vi "Select Players Dialog-old.vi"(8 "error in (no error)":errorcluster, 11 "Reversi in":refnum<class "Reversi.lvclass">) -> (0 "error out":errorcluster, 3 "Reversi out":refnum<class "Reversi.lvclass">)   [LabVIEW 2021, in "Reversi.lvlib" / "Reversi.lvclass"]
uses:
  Reversi.lvclass
  Reversi.lvclass/Reversi.ctl
  aa9f3d6a-4b9f-455d-bcc5-b1d428e522bf.vi
  edd00b8c-893c-4bab-b4e2-fb96aafeb1a1.vi
  <vilib>/Comparison/Equal/Equal Functor/Equal Functor.lvclass
panel:
  in  "White":string(combo)
  in  "Black":string(combo)
  in  "Start":bool
  # "Choose Players"
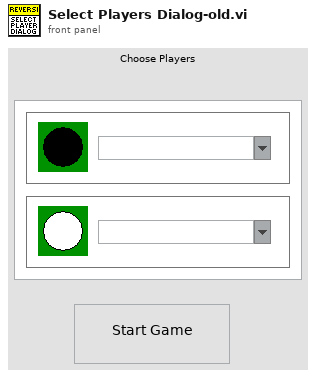
[diagram p1: front panel]
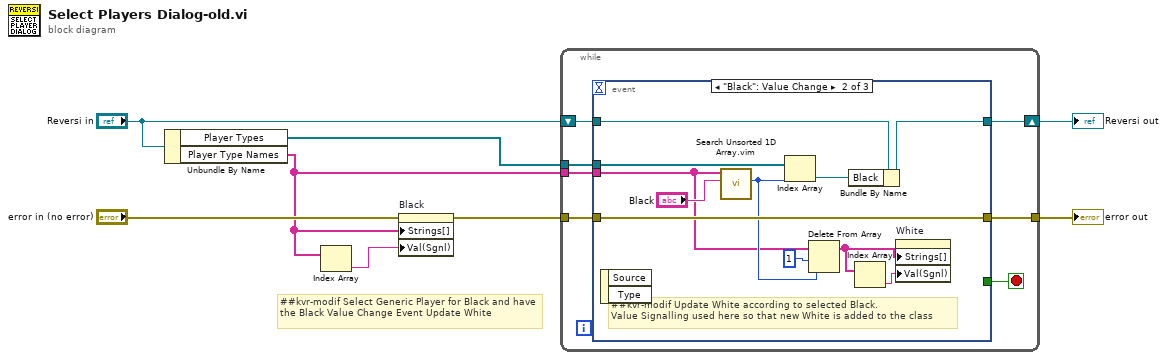
[diagram p0: block diagram]
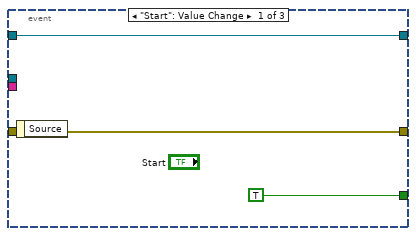
[diagram p2: hidden frame]
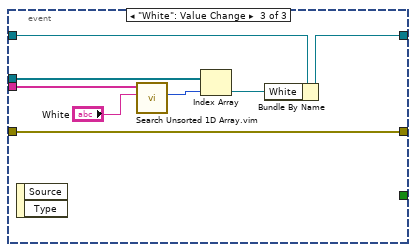
[diagram p3: hidden frame]
diagram:
  # "##kvr-modif Select Generic Player for Black and have the Black Value Change Event Update White"
  n1 = Unbundle By Name("Reversi in") -> ("Player Types"=w4:refnum<class "Player.lvclass">[], "Player Type Names"=w2:string[])
  n2 = Index Array(array=w2) -> (element=w1:string)  [unwired: 1 in]
  n3 = property on="Black" class="CmbBox"(error in="error in (no error)", "Strings[]"=w2, "Val(Sgnl)"=w1) -> (error out=w7:errorcluster)  [unwired: 1 in, 1 out]
  n4 = while {
    shift-right: [w13] -> w8
    shift-left: "Reversi in" -> [w15]
    tunnel: w4 -> [w11]
    tunnel: w2 -> [w12]
    tunnel: w7 -> [w10]
    tunnel: [w9] -> w5
    stop <- w14 stop-if-true
    n5 = event shown="[1] \"Black\": Value Change" {
      selector: _ -> [_ _ _]
      dyn-events: _ -> [_ _ _]
      timeout: _ -> [_ _ _]
      tunnel: w15 -> [w18 w26 w33]
      tunnel: [TRUE _ _] -> w14
      tunnel: [w18 w27 w34] -> w13
      tunnel: w12 -> [_ w19 w37]
      tunnel: w11 -> [_ w28 w36]
      tunnel: w10 -> [w16 w24 w30]
      tunnel: [w16 w24 w30] -> w9
      event "Start": Value Change {
        n6 = event-data() -> ()  [unwired: 1 in, 1 out]
      }
      event "Black": Value Change {
        # "##kvr-modif Update White according to selected Black.\nValue Signalling used here so that new White is added to the class"
        n7 = event-data() -> ()  [unwired: 1 in, 2 out]
        n8 = call "Search Unsorted 1D Array.vim"("element"="Black", "unsorted 1D array"=w19) -> ("index of element"=w20:i32)  [unwired: 9 in]
        n9 = Index Array(array=w28, index=w20) -> (element=w25:refnum<class "Player.lvclass">)
        n10 = Delete From Array(array=w19, length=1, index=w20) -> (array with subset deleted=w22:string[])  [unwired: 1 out]
        n11 = Bundle By Name(cluster=w26, "Black"=w25) -> (w27:refnum<class "Reversi.lvclass">)
        n12 = Index Array(array=w22) -> (element=w23:string)  [unwired: 1 in]
        n13 = property on="White" class="CmbBox"("Strings[]"=w22, "Val(Sgnl)"=w23) -> ()  [unwired: 2 in, 2 out]
      }
      event "White": Value Change {
        n14 = event-data() -> ()  [unwired: 1 in, 2 out]
        n15 = call "Search Unsorted 1D Array.vim"("element"="White", "unsorted 1D array"=w37) -> ("index of element"=w35:i32)  [unwired: 9 in]
        n16 = Index Array(array=w36, index=w35) -> (element=w32:refnum<class "Player.lvclass">)
        n17 = Bundle By Name(cluster=w33, "White"=w32) -> (w34:refnum<class "Reversi.lvclass">)
      }
    }
  }
  "error out" <- w5
  "Reversi out" <- w8
